vi "permute_axes.vi"(10 "Axis mapping":i32[](array[numeric])=[0, 1, 2, 3, 4, 5], 11 "Pulse count":i16[](array[numeric])) -> (3 "Result":i16[](array[numeric]))   [LabVIEW 2013]
panel:
  # "This VI lets us remap the axes in software if \nfor some reason the hardware mapping\ndoesn't correspond to the kinematic model."
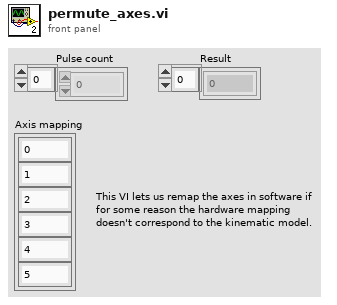
[diagram p1: front panel]
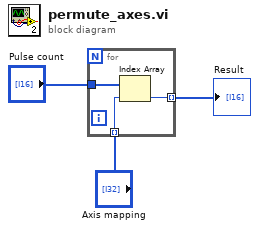
[diagram p0: block diagram]
diagram:
  n1 = for {
    tunnel: "Pulse count" -> [w6]
    tunnel: [w5] -> w2 mode=indexing
    tunnel: "Axis mapping" -> [w4] mode=indexing
    n2 = Index Array(array=w6, index=w4) -> (element=w5:i16)
  }
  "Result" <- w2
